vi "User data.vi"(0 "Operator Name":string="ID-0", 3 "Factory Name":string="EQD") -> (7 "refnum out":refnum<file>, 10 "error out":errorcluster)   [LabVIEW 2018]
uses:
  Global textParse.vi
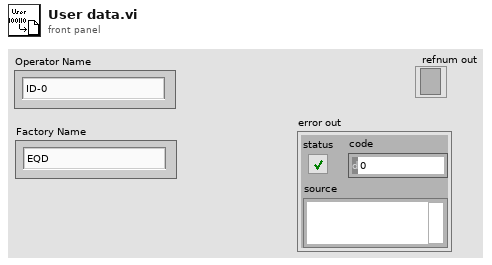
[diagram p1: front panel]
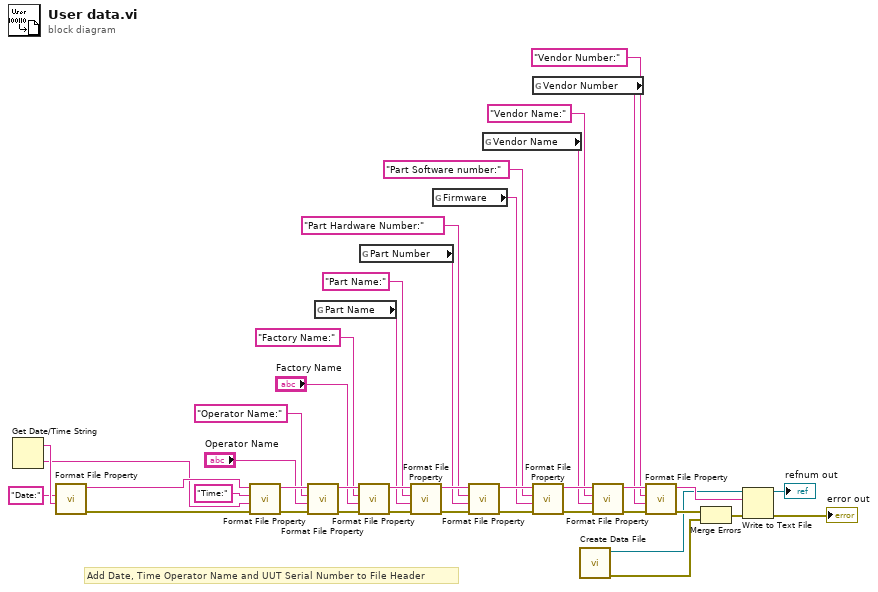
[diagram p0: block diagram]
diagram:
  # "Add Date, Time Operator Name and UUT Serial Number to File Header"
  n1 = Get Date/Time String() -> (date string=w28:string, time string=w16:string)  [unwired: 3 in]
  n2 = call "Format File Property.vi"("File Property Value"=w28, "File Property Name"="Date:") -> ("Error Out"=w24:errorcluster, "String out"=w27:string)  [unwired: 8 in]
  n3 = call "Format File Property.vi"("Error In"=w24, "File Property Value"=w16, "File Property Name"="Time:", "String in"=w27) -> ("Error Out"=w25:errorcluster, "String out"=w26:string)  [unwired: 6 in]
  n4 = call "Format File Property.vi"("Error In"=w25, "File Property Value"="Operator Name", "File Property Name"="Operator Name:", "String in"=w26) -> ("Error Out"=w23:errorcluster, "String out"=w22:string)  [unwired: 6 in]
  n5 = global read "Global textParse.vi" "Part Name"() -> (w12:string)
  n6 = call "Format File Property.vi"("Error In"=w23, "File Property Value"="Factory Name", "File Property Name"="Factory Name:", "String in"=w22) -> ("Error Out"=w14:errorcluster, "String out"=w15:string)  [unwired: 6 in]
  n7 = global read "Global textParse.vi" "Part Number"() -> (w30:string)
  n8 = call "Format File Property.vi"("Error In"=w14, "File Property Value"=w12, "File Property Name"="Part Name:", "String in"=w15) -> ("Error Out"=w13:errorcluster, "String out"=w37:string)  [unwired: 6 in]
  n9 = global read "Global textParse.vi" "Firmware"() -> (w34:string)
  n10 = call "Format File Property.vi"("Error In"=w13, "File Property Value"=w30, "File Property Name"="Part Hardware Number:", "String in"=w37) -> ("Error Out"=w29:errorcluster, "String out"=w38:string)  [unwired: 6 in]
  n11 = global read "Global textParse.vi" "Vendor Name"() -> (w35:string)
  n12 = global read "Global textParse.vi" "Vendor Number"() -> (w36:string)
  n13 = call "Format File Property.vi"("Error In"=w29, "File Property Value"=w34, "File Property Name"="Part Software number:", "String in"=w38) -> ("Error Out"=w31:errorcluster, "String out"=w39:string)  [unwired: 6 in]
  n14 = call "Create Data File.vi"() -> ("Error Out"=w17:errorcluster, "File Refnum"=w19:refnum<file>)  [unwired: 10 in]
  n15 = call "Format File Property.vi"("Error In"=w31, "File Property Value"=w35, "File Property Name"="Vendor Name:", "String in"=w39) -> ("Error Out"=w32:errorcluster, "String out"=w40:string)  [unwired: 6 in]
  n16 = call "Format File Property.vi"("Error In"=w32, "File Property Value"=w36, "File Property Name"="Vendor Number:", "String in"=w40) -> ("Error Out"=w33:errorcluster, "String out"=w41:string)  [unwired: 6 in]
  n17 = Merge Errors(w33, w17) -> (w18:errorcluster)
  n18 = Write to Text File(file (use dialog)=w19, text=w41, error in=w18) -> (refnum out=→"refnum out":refnum<file>, error out=→"error out":errorcluster)  [unwired: 1 in, 1 out]
